vi "CTRE_PigeonIMU_SetCompass.vi"(8 "error in (no error)":errorcluster, 10 "Offset":dbl, 11 "PigeonIMUDevRef":T1={"DeviceStatus"={"status"=FALSE, "code"=0, "source"=""}, "Device Number"=0, "Type"=352321536, "Device ID"=0, "Handle"=0, "UsageFrame"=0, "Library Path"=path ""} {"Type" items=["CAN"=352321536, "TalonSRX"=33554432]}) -> (0 "error out":errorcluster, 3 "PigeonIMUDevRef":T1={"DeviceStatus"={"status"=FALSE, "code"=0, "source"=""}, "Device Number"=0, "Type"=352321536, "Device ID"=0, "Handle"=0, "UsageFrame"=0, "Library Path"=path ""} {"Type" items=["CAN"=352321536, "TalonSRX"=33554432]})   [LabVIEW 2016]
uses:
  <vilib>/Rock Robotics/WPI/ThirdParty/Sensors/Pigeon IMU/CTRE_PigeonIMU_DeviceRef.ctl
  <vilib>/Rock Robotics/WPI/ThirdParty/Sensors/Pigeon IMU/CTRE_PigeonIMU_ConnectionType.ctl
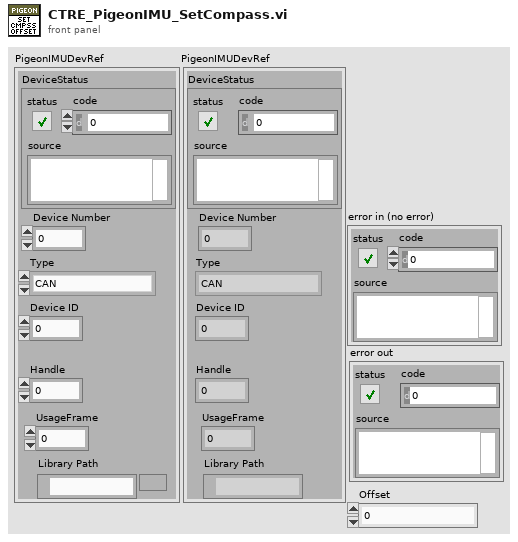
[diagram p1: front panel]
types:
  T1 = typedef "CTRE_PigeonIMU_DeviceRef.ctl" = cluster{"DeviceStatus":errorcluster, "Device Number":u8, "Type":T2, "Device ID":u32, "Handle":u64, "UsageFrame":u32, "Library Path":path}
  T2 = typedef "CTRE_PigeonIMU_ConnectionType.ctl" = u32
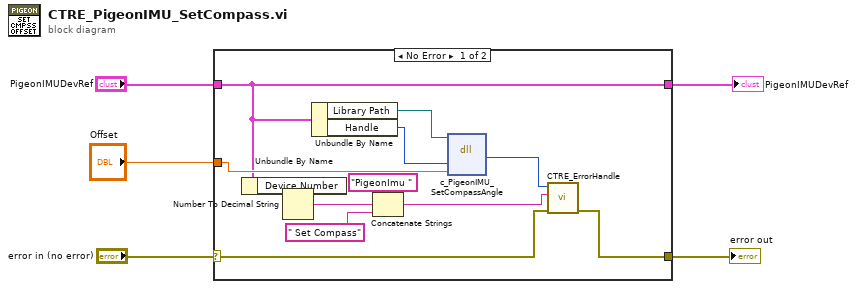
[diagram p0: block diagram]
diagram:
  n1 = case shown="No Error" "error in (no error)" {
    selector: "error in (no error)" -> [w9 w18]
    tunnel: [w8 w18] -> w4
    tunnel: [w6 w19] -> w2
    tunnel: "PigeonIMUDevRef" -> [w6 w19]
    tunnel: "Offset" -> [w15 _]
    frame No Error {
      n2 = Unbundle By Name(w6) -> ("Device Number"=w11:u8)
      n3 = Number To Decimal String(number=w11) -> (decimal integer string=w12:string)  [unwired: 1 in]
      n4 = Unbundle By Name(w6) -> ("Library Path"=w17:path, "Handle"=w16:u64)
      n5 = Concatenate Strings("PigeonImu " ("string"), w12, " Set Compass" ("string")) -> (w7:string)
      n6 = dll-call lib="?" fn="c_PigeonIMU_SetCompassAngle"(path in=w17, "handle"=w16, "angleDeg"=w15) -> ("return type"=w10:i32)  [unwired: 4 in, 2 out]
      n7 = call <vilib>:"CTRE_ErrorHandle.vi"("error in"=w9, "origin"=w7, "code"=w10) -> ("error out"=w8:errorcluster)  [unwired: 8 in]
    }
    frame Error {
    }
  }
  "PigeonIMUDevRef" <- w2
  "error out" <- w4
